vi "Refresh All Feeds.vi"(8 "error in":errorcluster) -> (0 "error out":errorcluster, 3 "refreshed feeds":string[](array[string]))   [LabVIEW 2014, in "NIPM_API.lvlib"]
doc: "Refreshes NI Package Manager with data from all registered feeds.\n\nNote: You should refresh after adding/removing packages from feeds, so that NI Package Manager will update with the latest feed and package data.\n\nOUTPUT(s)\n<B>Refreshed feeds</B>: Outputs a 1D array containing the names of all refreshed feeds."
uses:
  NIPM_API.lvlib
panel:
  out "command line standard output":string
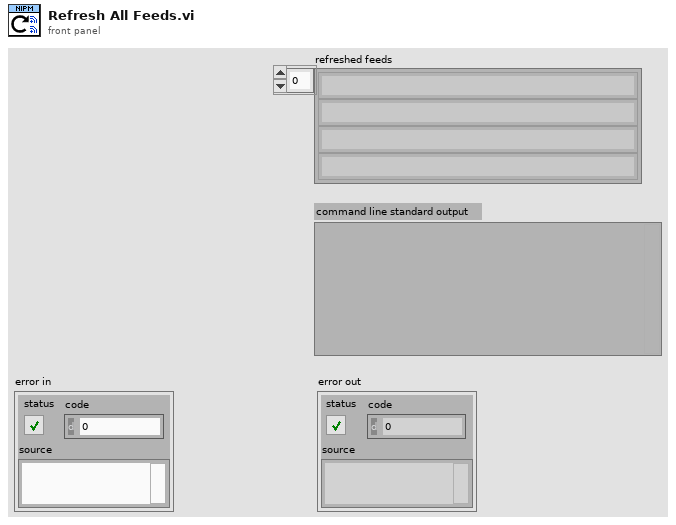
[diagram p1: front panel]
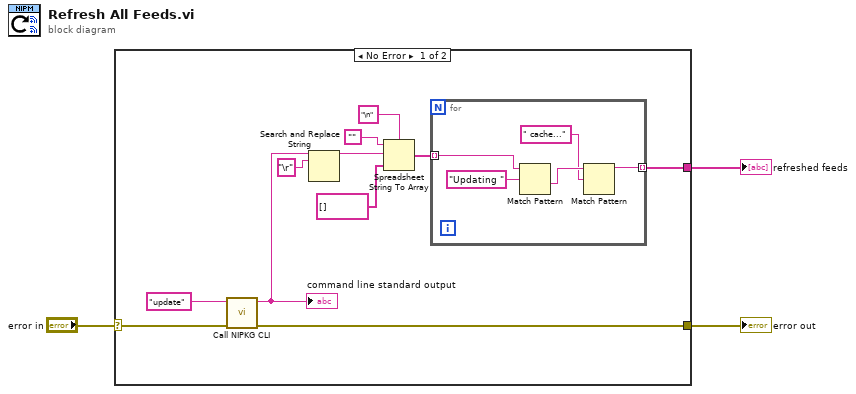
[diagram p0: block diagram]
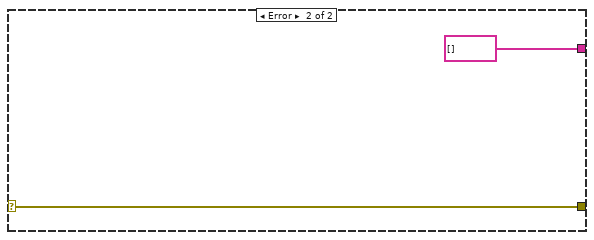
[diagram p2: hidden frame]
diagram:
  n1 = case shown="No Error" "error in" {
    selector: "error in" -> [w14 w21]
    tunnel: [w12 w21] -> w2
    tunnel: [w4 string[] []] -> w1
    frame No Error {
      n2 = call "Call NIPKG CLI.vi"("error in (no error)"=w14, "command"="update" ("format string")) -> ("error out"=w12:errorcluster, "command line standard output"=w11:string)  [unwired: 8 in]
      "command line standard output" <- w11
      n3 = Search and Replace String(input string=w11, search string="\r") -> (result string=w9:string)  [unwired: 6 in, 3 out]
      n4 = Spreadsheet String To Array(delimiter (Tab)="\n", format string="", spreadsheet string=w9, array type (2D Dbl)=string[] []) -> (array=w5:string[])
      n5 = for {
        tunnel: w5 -> [w18] mode=indexing
        tunnel: [w15] -> w4 mode=indexing
        n6 = Match Pattern(string=w18, regular expression="Updating ") -> (after substring=w17:string)  [unwired: 1 in, 3 out]
        n7 = Match Pattern(string=w17, regular expression=" cache...") -> (before substring=w15:string)  [unwired: 1 in, 3 out]
      }
    }
    frame Error {
    }
  }
  "error out" <- w2
  "refreshed feeds" <- w1
